vi "example2.vi"() -> ()   [LabVIEW 2020]
uses:
  ControlCAN/ControlCAN.lvlib
  ControlCAN/ControlCAN.llb/VCI_CAN_OBJ.ctl
panel:
  in  "Buffer":T1[](array[typedef])
  out "Recieve 3":T1[](array[typedef])
  out "Recieve 2":T1[](array[typedef])
  out "子字符串":string
  in  "DevType 2":u32(ring)=2 items=["USB-CAN"=2, "USB-CAN2"=3]
  in  "DevType":T2=2 items=["USB-CAN"=2, "USB-CAN2"=3]
  in  "DevType":u32(ring)=2 items=["USB-CAN"=2, "USB-CAN2"=3]
  in  "等待时间（毫秒）":fxp<+,32,32>
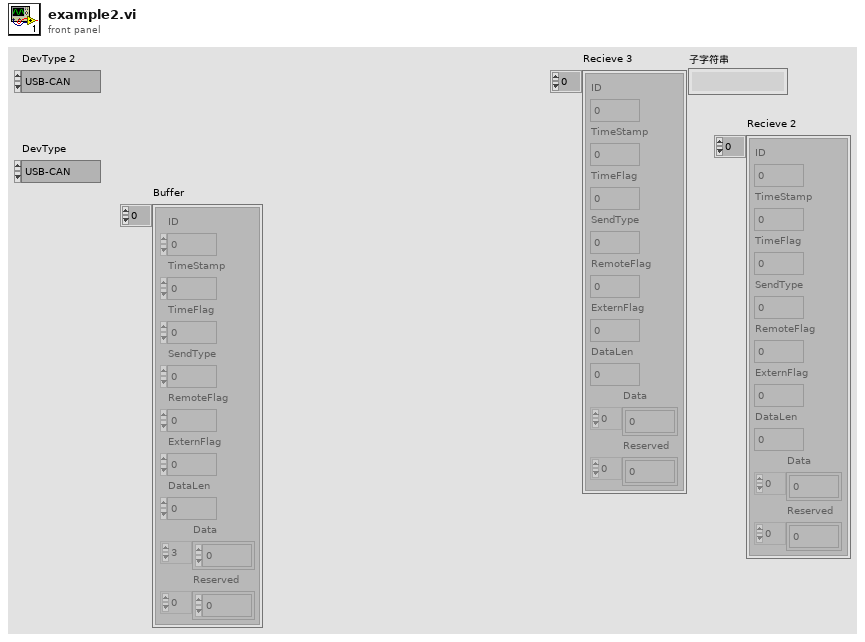
[diagram p1: front panel]
types:
  T1 = typedef "ControlCAN.lvlib/VCI_CAN_OBJ.ctl" = cluster{"ID":u32, "TimeStamp":u32, "TimeFlag":u8, "SendType":u8, "RemoteFlag":u8, "ExternFlag":u8, "DataLen":u8, "Data":u8[], "Reserved":u8[]}
  T2 = typedef "控件 2.ctl" = u32
  T3 = cluster{"Recieve 3[0]":T1, "Recieve 3[1]":T1, "Recieve 3[2]":T1, "Recieve 3[3]":T1, "Recieve 3[4]":T1, "Recieve 3[5]":T1, "Recieve 3[6]":T1, "Recieve 3[7]":T1, "Recieve 3[8]":T1, "Recieve 3[9]":T1, "Recieve 3[10]":T1, "Recieve 3[11]":T1}
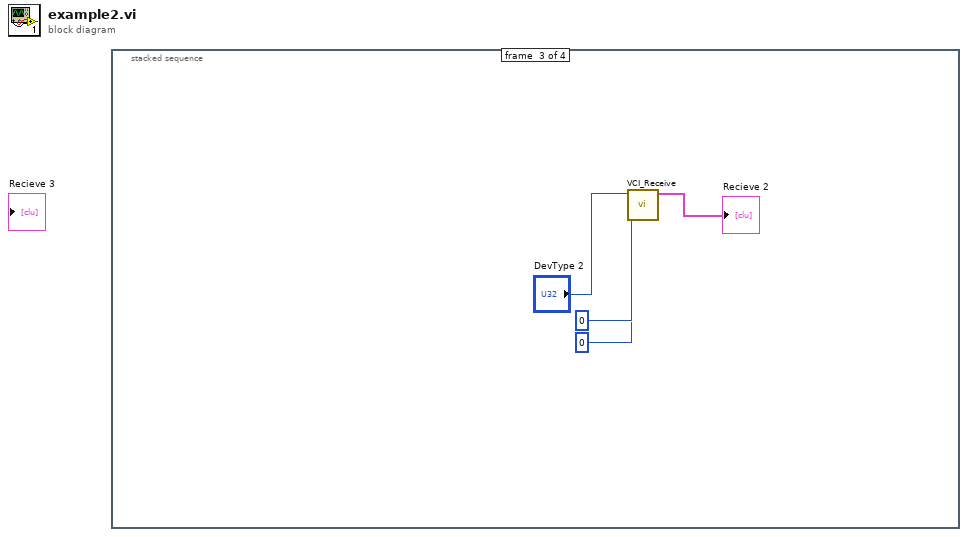
[diagram p0: block diagram]
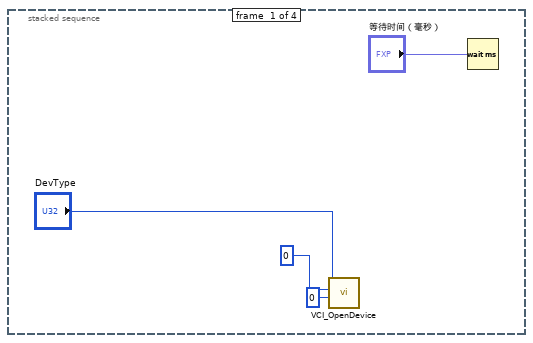
[diagram p2: hidden frame]
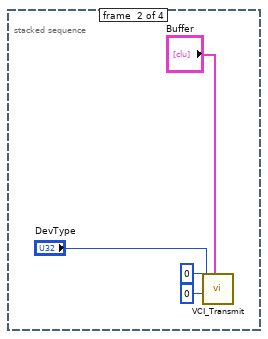
[diagram p3: hidden frame]
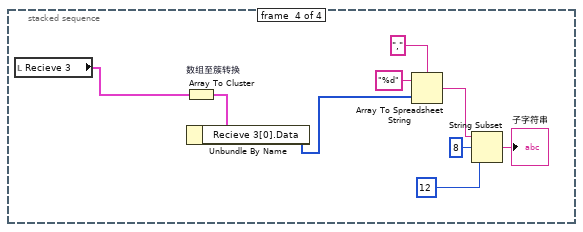
[diagram p4: hidden frame]
diagram:
  n1 = stacked-sequence {
    frame #0 {
      n2 = call "VCI_OpenDevice.vi"("Reserved"=u32 0, "DevIndex"=u32 0, "DevType"="DevType") -> ()  [unwired: 7 in, 2 out]
      n3 = Wait (ms)(milliseconds to wait="等待时间（毫秒）") -> ()  [unwired: 1 out]
    }
    frame #1 {
      n4 = call "VCI_Transmit.vi"("Buffer"="Buffer", "CANIndex"=u32 0, "DevIndex"=u32 0, "DevType"="DevType") -> ()  [unwired: 6 in, 2 out]
    }
    frame #2 {
      n5 = call "VCI_Receive.vi"("CANIndex"=u32 0, "DevIndex"=u32 0, "DevType"="DevType 2") -> ("Recieve"=→"Recieve 2":T1[])  [unwired: 7 in, 1 out]
    }
    frame #3 {
      n6 = local read "Recieve 3"() -> (w15:T1[])
      n7 = Array To Cluster "数组至簇转换"(array=w15) -> (cluster=w14:T3)
      n8 = Unbundle By Name(w14) -> ("Recieve 3[0].Data"=w13:u8[])
      n9 = Array To Spreadsheet String(delimiter (Tab)="," ("分隔符(Tab)"), array=w13, 3:"%d" ("格式字符串")) -> (spreadsheet string=w19:string)
      n10 = String Subset(string=w19, offset (0)=8 ("偏移量(0)"), length (rest)=12 ("长度（剩余）")) -> (substring=→"子字符串":string)
    }
  }
